vi "Shift Lidar.vi"(6 "XY":T1, 8 "Angle":dbl, 9 "X position":dbl, 10 "Y position":dbl, 11 "Resolution":dbl) -> (0 "PosY":dbl, 1 "Shifted X":dbl, 2 "Shifted Y":dbl, 3 "PosX":dbl)   [LabVIEW 2017]
uses:
  040-typeDefs/LidarPoint.ctl
  <vilib>/Analysis/coordinate.llb/2D Cartesian Coordinate Rotation (Scalar).vi
  <vilib>/Analysis/NI_AALPro.lvlib
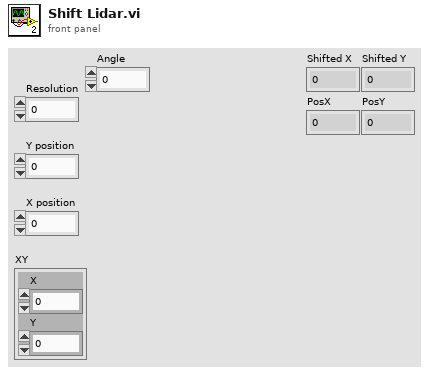
[diagram p1: front panel]
types:
  T1 = typedef "LidarPoint.ctl" = cluster{"X":dbl, "Y":dbl}
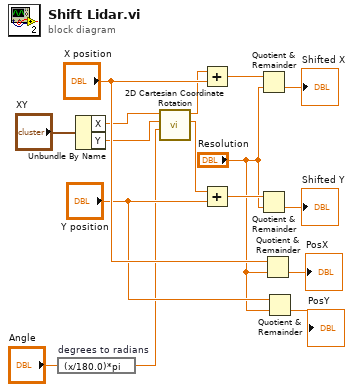
[diagram p0: block diagram]
diagram:
  n1 = expression code="(x/180.0)*pi" "degrees to radians"("Angle") -> (w2:dbl)
  n2 = Unbundle By Name("XY") -> ("X"=w6:dbl, "Y"=w4:dbl)
  n3 = call-poly <vilib>:"2D Cartesian Coordinate Rotation.vi"("theta"=w2, "y"=w4, "x"=w6) -> ("y out"=w3:dbl, "x out"=w5:dbl)  [unwired: 6 in, 1 out]
  n4 = Add(x=w5, y="X position") -> (x+y=w15:dbl)
  n5 = Add(x=w3, y="Y position") -> (x+y=w16:dbl)
  n6 = Quotient & Remainder(x=w15, y="Resolution") -> (floor(x/y)=→"Shifted X":dbl)  [unwired: 1 out]
  n7 = Quotient & Remainder(x=w16, y="Resolution") -> (floor(x/y)=→"Shifted Y":dbl)  [unwired: 1 out]
  n8 = Quotient & Remainder(x="X position", y="Resolution") -> (floor(x/y)=→"PosX":dbl)  [unwired: 1 out]
  n9 = Quotient & Remainder(x="Y position", y="Resolution") -> (floor(x/y)=→"PosY":dbl)  [unwired: 1 out]
